vi "q3 factorial.vi"(10 "n":dbl) -> (2 "n!":dbl)   [LabVIEW 2025]
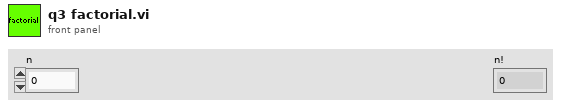
[diagram p1: front panel]
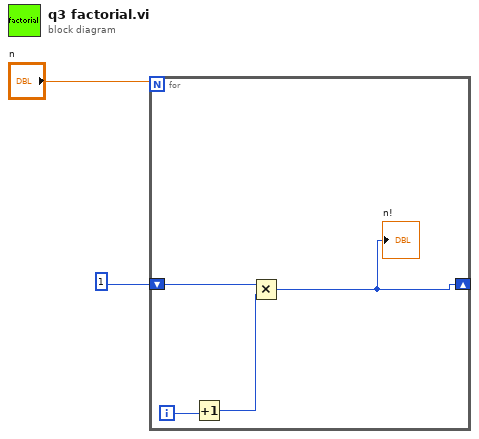
[diagram p0: block diagram]
diagram:
  n1 = for {
    N: "n" -> [_]
    shift-right: [w3] -> _
    shift-left: 1 -> [w4]
    i -> [w6]
    n2 = Increment(x=w6) -> (x+1=w5:i32)
    n3 = Multiply(x=w4, y=w5) -> (x*y=w3:i32)
    "n!" <- w3
  }
